vi "Set Common Doc Dir.vi"(10 "Common Doc Dir":string, 11 "Project XML Editor in":refnum<class "Project XML Editor.lvclass">) -> (3 "Project XML Editor out":refnum<class "Project XML Editor.lvclass">)   [LabVIEW 2018, in ".LVLIBP CD XML Updater.lvlib" / "Project XML Editor.lvclass"]
uses:
  Project XML Editor.lvclass
  Project XML Editor.lvclass/Project XML Editor.ctl
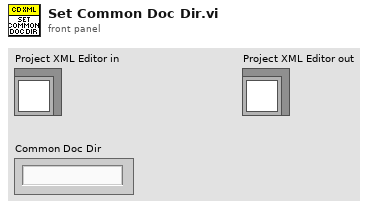
[diagram p1: front panel]
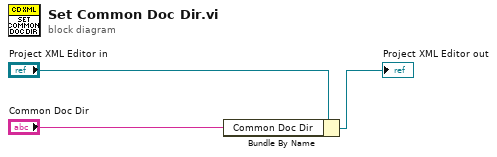
[diagram p0: block diagram]
diagram:
  n1 = Bundle By Name(cluster="Project XML Editor in", "Common Doc Dir"="Common Doc Dir") -> (→"Project XML Editor out":refnum<class "Project XML Editor.lvclass">)
